vi "Set Default.vi"(11 "Integer in":refnum<class "Integer.lvclass">) -> (3 "Integer out":refnum<class "Integer.lvclass">)   [LabVIEW 2022 SP3, in "Conditum.lvlib" / "Columns.lvlib" / "Integer.lvclass"]
uses:
  Integer.lvclass
  Integer.lvclass/Integer.ctl
  Type/Type.lvclass
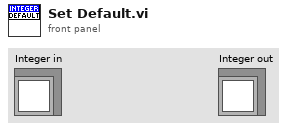
[diagram p1: front panel]
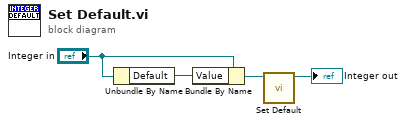
[diagram p0: block diagram]
diagram:
  n1 = Unbundle By Name("Integer in") -> ("Default"=w4:i64)
  n2 = Bundle By Name(cluster="Integer in", "Value"=w4) -> (w3:refnum<class "Integer.lvclass">)
  n3 = call-parent "Set Default.vi"("Type in"=w3) -> ("Type out"=→"Integer out":refnum<class "Integer.lvclass">)  [unwired: 10 in]
